vi "Lein stat2 read system status.vi"(0 "higher in hierarchy connected(T)":bool=TRUE, 7 "sys register":u16 format="%.0x", 11 "error in (no error)":errorcluster) -> (3 "Force NA":bool, 4 "Stopped":bool, 6 "Error":T2, 8 "Connected":bool, 10 "Task":T3, 13 "All status":T1, 14 "User bit":bool, 15 "error out":errorcluster)   [LabVIEW 2011]
uses:
  Stat2 system error.ctl
  Stat2 system task info.ctl
  Status any node.ctl
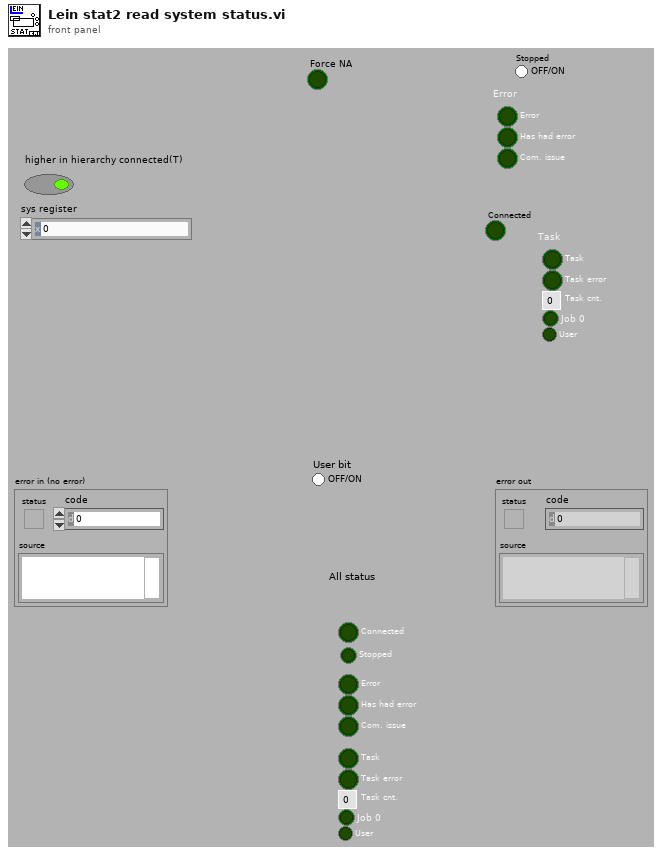
[diagram p1: front panel]
types:
  T1 = typedef "Status any node.ctl" = cluster{"Name":string, "Connected":bool, "Stopped":bool, "Error":T2, "Task":T3}
  T2 = typedef "Stat2 system error.ctl" = cluster{"Error":bool, "Has had error":bool, "Com. issue":bool}
  T3 = typedef "Stat2 system task info.ctl" = cluster{"Task":bool, "Task error":bool, "Task cnt.":u8, "Job 0":bool, "User":bool}
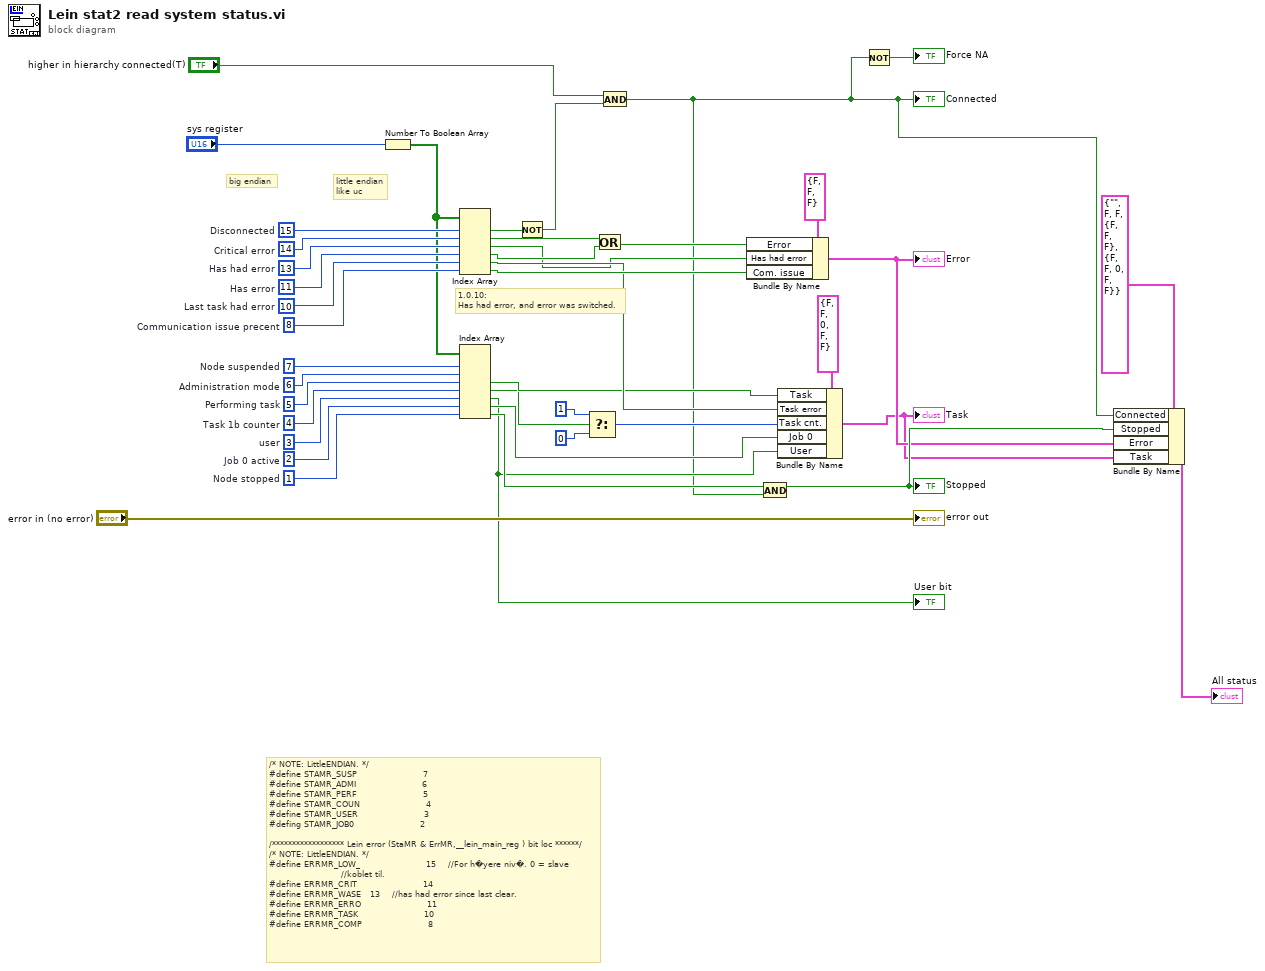
[diagram p0: block diagram]
diagram:
  w13 = 1  # Node stopped
  w14 = 2  # Job 0 active
  w30 = 3  # user
  w31 = 4  # Task 1b counter
  w32 = 5  # Performing task
  w33 = 6  # Administration mode
  w34 = 7  # Node suspended
  w36 = 8  # Communication issue precent
  w37 = 10  # Last task had error
  w38 = 11  # Has error
  w39 = 13  # Has had error
  w40 = 14  # Critical error
  w41 = 15  # Disconnected
  # "1.0.10:\nHas had error, and error was switched."
  # "/* NOTE: LittleENDIAN. */\n#define STAMR_SUSP                      7\n#define STAMR_ADMI                      6\n#define STAMR_PERF                      5\n#define STAMR_COUN                      4\n#define STAMR_USER                      3\n#defing STAMR_JOB0                      2\n\n/****************** Lein error (StaMR & ErrMR,__lein_main_reg ) bit loc ******/\n/* NOTE: LittleENDIAN. */\n#define ERRMR_LOW_                      15    //For h�yere niv�. 0 = slave\n                        //koblet til.\n#define ERRMR_CRIT                      14\n#define ERRMR_WASE\t\t\t13    //has had error since last clear.\n#define ERRMR_ERRO                      11\n#define ERRMR_TASK                      10\n#define ERRMR_COMP                      8"
  # "little endian\nlike uc"
  # "big endian"
  n1 = Number To Boolean Array(number="sys register") -> (Boolean array=w35:bool[])
  n2 = Index Array(array=w35, index #1=w41, index #2=w40, index #3=w39, index #4=w38, index #5=w37, index #6=w36) -> (element #1=w29:bool, element #2=w26:bool, element #3=w7:bool, element #4=w8:bool, element #5=w21:bool, element #6=w23:bool)
  n3 = Index Array(array=w35, index #1=w34, index #2=w33, index #3=w32, index #4=w31, index #5=w30, index #6=w14, index #7=w13) -> (element #3=w18:bool, element #4=w17:bool, element #5=w9:bool, element #6=w10:bool, element #7=w12:bool)  [unwired: 2 out]
  "User bit" <- w9
  n4 = Not(x=w29) -> (.not. x?=w28:bool)
  n5 = Select(t=u8 1 ("Task counter"), s=w17, f=u8 0 ("Task counter")) -> (s? t:f=w16:u8)
  n6 = Or(x=w26, y=w8) -> (x .or. y?=w24:bool)
  n7 = And(x="higher in hierarchy connected(T)", y=w28) -> (x .and. y?=w4:bool)
  "Connected" <- w4
  n8 = Bundle By Name(cluster=T2 {"Error"=FALSE, "Has had error"=FALSE, "Com. issue"=FALSE} ("Stat2 system error"), "Error"=w24, "Has had error"=w7, "Com. issue"=w23) -> (w2:T2)
  "Error" <- w2
  n9 = And(x=w12, y=w4) -> (x .and. y?=w3:bool)
  "Stopped" <- w3
  n10 = Bundle By Name(cluster=T3 {"Task"=FALSE, "Task error"=FALSE, "Task cnt."=0, "Job 0"=FALSE, "User"=FALSE} ("Stat2 system  task info"), "Task"=w18, "Task error"=w21, "Task cnt."=w16, "Job 0"=w10, "User"=w9) -> (w1:T3)
  "Task" <- w1
  n11 = Not(x=w4) -> (.not. x?=→"Force NA":bool)
  n12 = Bundle By Name(cluster=T1 {"Name"="", "Connected"=FALSE, "Stopped"=FALSE, "Error"={"Error"=FALSE, "Has had error"=FALSE, "Com. issue"=FALSE}, "Task"={"Task"=FALSE, "Task error"=FALSE, "Task cnt."=0, "Job 0"=FALSE, "User"=FALSE}} ("All status"), "Connected"=w4, "Stopped"=w3, "Error"=w2, "Task"=w1) -> (→"All status":T1)
  "error out" <- "error in (no error)"
